vi "WhichVIsShouldRegenerate.vi"(8 "DoAllOfThem":bool, 10 "CommandTemplatesFolder":path=path "C:/Users/competition/Documents/LabVIEW Data/Projects/xml-auto-routine/CreateCommands/CommandTemplates", 11 "LastModifiedDatesFolder":path=path "C:/Users/competition/Documents/LabVIEW Data/Projects/xml-auto-routine/CreateCommands") -> (0 "New VI":bool, 2 "iniRefecence":T1, 3 "VINames":string[](array[string]))   [LabVIEW 2020]
uses:
  <vilib>/Utility/config.llb/Config Data RefNum.ctl
  <vilib>/Utility/config.llb/Read Key (String).vi
  <vilib>/Utility/config.llb/NI_LVConfig.lvlib
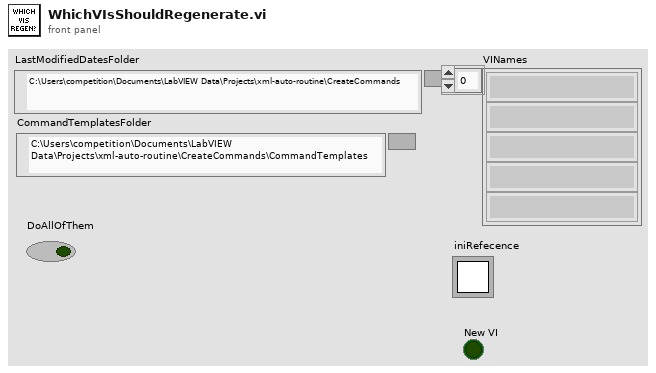
[diagram p1: front panel]
types:
  T1 = typedef "NI_LVConfig.lvlib/Config Data RefNum.ctl" = refnum<k1>
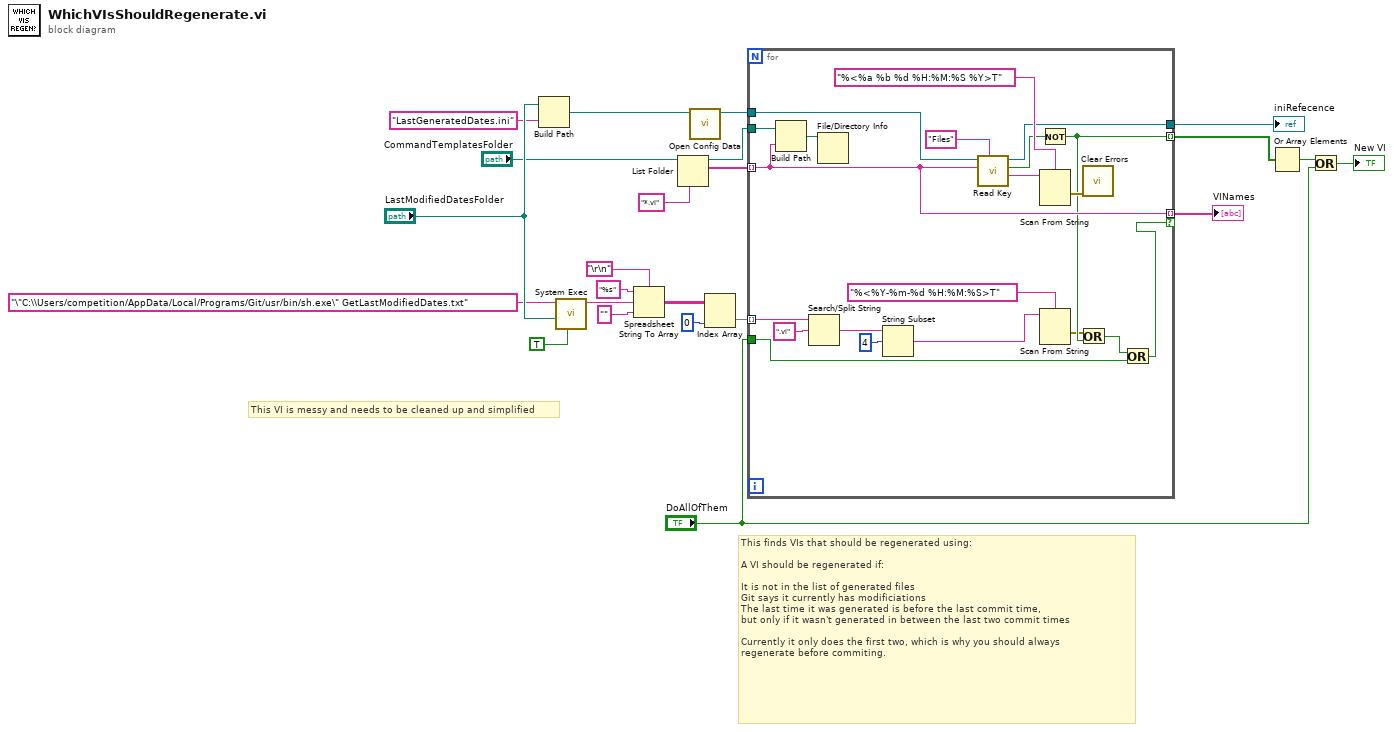
[diagram p0: block diagram]
diagram:
  # "This VI is messy and needs to be cleaned up and simplified"
  # "This finds VIs that should be regenerated using:\n\nA VI should be regenerated if:\n\nIt is not in the list of generated files\nGit says it currently has modificiations\nThe last time it was generated is before the last commit time,\nbut only if it wasn't generated in between the last two commit times\n\nCurrently it only does the first two, which is why you should always\nregenerate before commiting."
  n1 = Build Path(base path="LastModifiedDatesFolder", name or relative path="LastGeneratedDates.ini") -> (appended path=w20:path)
  n2 = call <vilib>:"System Exec.vi"("run minimized? (F)"=TRUE, "working directory"="LastModifiedDatesFolder", "command line"="\"C:\\Users/competition/AppData/Local/Programs/Git/usr/bin/sh.exe\" GetLastModifiedDates.txt") -> ("standard output"=w5:string)  [unwired: 5 in, 3 out]
  n3 = Spreadsheet String To Array(delimiter (Tab)="\r\n", format string="%s", spreadsheet string=w5, array type (2D Dbl)="" ("format string")) -> (array=w2:string[][])
  n4 = List Folder(path="CommandTemplatesFolder", pattern="*.vi") -> (path out=w17:path, filenames=w18:string[])  [unwired: 2 in, 2 out]
  n5 = call <vilib>:"Open Config Data.vi"("configuration file path"=w20) -> ("refnum"=w16:T1)  [unwired: 8 in, 2 out]
  n6 = Index Array(array=w2, index (col)=0 ("disabled index (col)")) -> (element=w13:string[])  [unwired: 1 in]
  n7 = for {
    tunnel: w18 -> [w38] mode=indexing
    tunnel: w17 -> [w40]
    tunnel: w16 -> [w39]
    tunnel: [w38] -> w15 mode=indexing if=w24
    tunnel: [w37] -> w14
    tunnel: w13 -> [w34] mode=indexing
    tunnel: "DoAllOfThem" -> [w33]
    tunnel: [w32] -> w12 mode=indexing
    n8 = Build Path(base path=w40, name or relative path=w38) -> (appended path=w41:path)
    n9 = Search/Split String(string=w34, search string/char (-)=".vi") -> (match + rest of string=w30:string)  [unwired: 1 in, 2 out]
    n10 = File/Directory Info(path=w41) -> ()  [unwired: 1 in, 7 out]
    n11 = String Subset(string=w30, offset (0)=4) -> (substring=w29:string)  [unwired: 1 in]
    n12 = call-poly <vilib>:"Read Key.vi"("section"="Files", "key"=w38, "refnum"=w39) -> ("value"=w44:string, "found?"=w35:bool, "refnum out"=w37:T1)  [unwired: 5 in, 1 out]
    n13 = Not(x=w35) -> (.not. x?=w32:bool)
    n14 = Scan From String(format string="%<%a %b %d %H:%M:%S %Y>T", input string=w44) -> (error out=w36:errorcluster)  [unwired: 4 in, 2 out]
    n15 = Scan From String(format string="%<%Y-%m-%d %H:%M:%S>T", input string=w29) -> (error out=w27:errorcluster)  [unwired: 4 in, 2 out]
    n16 = Or(x=w27, y=w32) -> (x .or. y?=w25:bool)
    n17 = call <vilib>:"Clear Errors.vi"("error in (no error)"=w36) -> ()  [unwired: 5 in, 2 out]
    n18 = Or(x=w25, y=w33) -> (x .or. y?=w24:bool)
  }
  "VINames" <- w15
  "iniRefecence" <- w14
  n19 = Or Array Elements(Boolean array=w12) -> (logical OR=w11:bool)
  n20 = Or(x=w11, y="DoAllOfThem") -> (x .or. y?=→"New VI":bool)
